vi "QueryPerformanceCounter.vi"() -> (0 "counter":i64)   [LabVIEW 2009]
uses:
  kernel32.dll
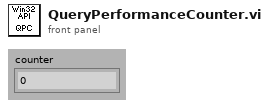
[diagram p1: front panel]
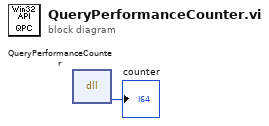
[diagram p0: block diagram]
diagram:
  n1 = dll-call lib="kernel32.dll" fn="QueryPerformanceCounter"() -> ("PerformanceCount"=→"counter":i64)  [unwired: 3 in, 4 out]
